vi "MoveUp.vi"(0 "Grids In":i32[][](array[numeric])) -> (1 "Grids Out":i32[][](array[numeric]), 2 "Score":i32, 3 "Moved?":bool)   [LabVIEW 2018]
doc: "Move grids up."
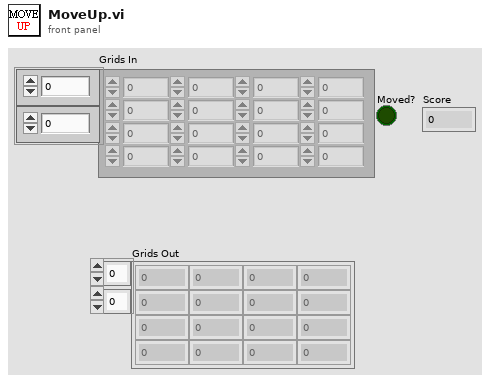
[diagram p1: front panel]
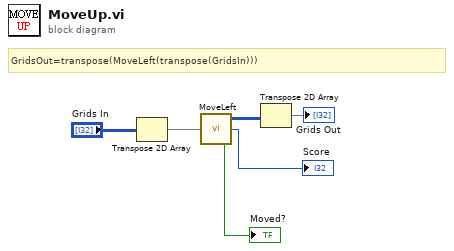
[diagram p0: block diagram]
diagram:
  # "GridsOut=transpose(MoveLeft(transpose(GridsIn)))"
  n1 = Transpose 2D Array(2D array="Grids In") -> (transposed array=w5:i32[][])
  n2 = call "MoveLeft.vi"("Grids In"=w5) -> ("Grid Out"=w4:i32[][], "Score"=→"Score":i32, "Moved?"=→"Moved?":bool)
  n3 = Transpose 2D Array(2D array=w4) -> (transposed array=→"Grids Out":i32[][])
